vi "Create Tasks.vi"(8 "error in":errorcluster, 11 "6509 in":refnum<class "6509.lvclass">) -> (0 "error out":errorcluster, 3 "6509 out":refnum<class "6509.lvclass">)   [LabVIEW 2019, in "6509.lvlib" / "6509.lvclass"]
uses:
  Library/6509.lvclass
  C:/Users/Public/Documents/Development/builds/Instruments/Instruments.lvlibp/Library/Instruments.lvclass
  C:/Users/Public/Documents/Development/builds/Instruments/DIG_IO.lvlibp/Library/DIG_IO.lvclass
  Library/6509.lvclass/6509.ctl
  builds/Instruments/Instruments.lvlibp/Accessors/Read Resource.vi
  builds/Instruments/DIG_IO.lvlibp/Accessors/Read IO_Mode.vi
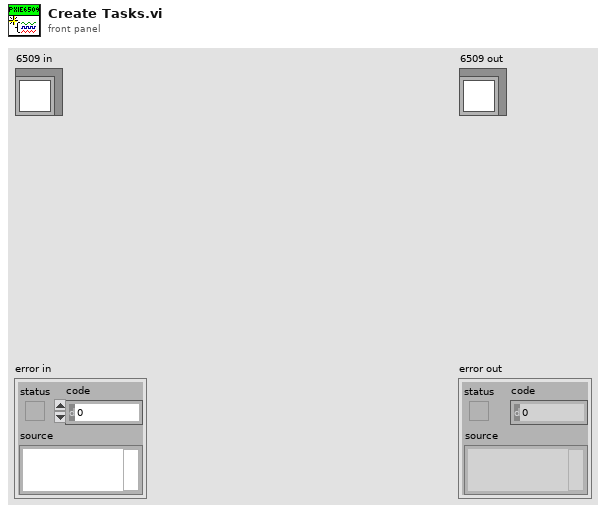
[diagram p1: front panel]
types:
  T1 = typedef "DIG_IO.lvlibp/DIG_IO.lvclass/IO Mode.ctl" = enum16{"IO", "IN", "OUT"}
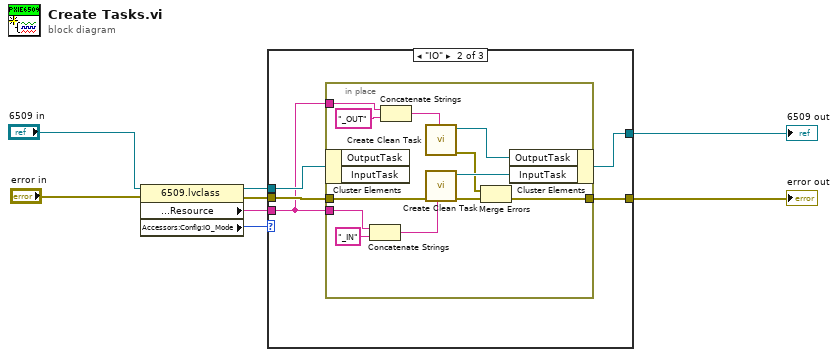
[diagram p0: block diagram]
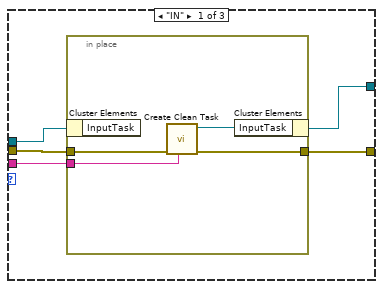
[diagram p2: hidden frame]
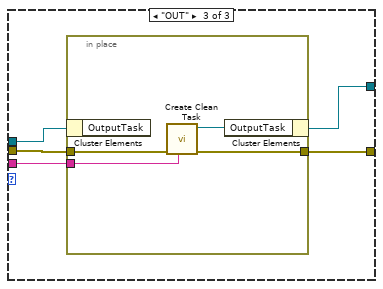
[diagram p3: hidden frame]
diagram:
  n1 = property class="6509.lvclass"(reference="6509 in", error in="error in") -> (reference out=w6:refnum<class "6509.lvclass">, error out=w4:errorcluster, "Accessors:Configuration:Resource"=w7:string, "Accessors:Config:IO_Mode"=w8:T1)
  n2 = case shown="\"IO\"" w8 {
    tunnel: w7 -> [w10 w18 w36]
    tunnel: w6 -> [w13 w22 w39]
    tunnel: [w12 w21 w38] -> w5
    tunnel: w4 -> [w11 w20 w37]
    tunnel: [w9 w19 w35] -> w3
    frame "IN" {
      n3 = in-place {
        in-place-border: w11 -> [w16]
        in-place-border: w10 -> [w15]
        in-place-border: [w14] -> w9
        n4 = in-place-cluster #1(w13) -> ()  [unwired: 1 out]
        n5 = call "Create Clean Task.vi"("Task Name"=w15, "error in (no error)"=w16) -> ("error out"=w14:errorcluster, "task out"=w17:refnum<k21>)  [unwired: 8 in]
        n6 = in-place-cluster #1("InputTask"=w17) -> (w12:refnum<class "6509.lvclass">)
      }
    }
    frame "IO" {
      n7 = in-place {
        in-place-border: w20 -> [w33]
        in-place-border: w18 -> [w32]
        in-place-border: [w25] -> w19
        in-place-border: w18 -> [w28]
        n8 = in-place-cluster #2(w22) -> ()  [unwired: 2 out]
        n9 = Concatenate Strings(w32, "_IN" ("string")) -> (w30:string)
        n10 = Concatenate Strings(w28, "_OUT" ("string")) -> (w27:string)
        n11 = call "Create Clean Task.vi"("Task Name"=w27) -> ("error out"=w23:errorcluster, "task out"=w26:refnum<k21>)  [unwired: 9 in]
        n12 = call "Create Clean Task.vi"("Task Name"=w30, "error in (no error)"=w33) -> ("error out"=w24:errorcluster, "task out"=w34:refnum<k21>)  [unwired: 8 in]
        n13 = Merge Errors(w23, w24) -> (w25:errorcluster)
        n14 = in-place-cluster #2("OutputTask"=w26, "InputTask"=w34) -> (w21:refnum<class "6509.lvclass">)
      }
    }
    frame "OUT" {
      n15 = in-place {
        in-place-border: w37 -> [w42]
        in-place-border: w36 -> [w41]
        in-place-border: [w40] -> w35
        n16 = in-place-cluster #3(w39) -> ()  [unwired: 1 out]
        n17 = call "Create Clean Task.vi"("Task Name"=w41, "error in (no error)"=w42) -> ("error out"=w40:errorcluster, "task out"=w43:refnum<k21>)  [unwired: 8 in]
        n18 = in-place-cluster #3("OutputTask"=w43) -> (w38:refnum<class "6509.lvclass">)
      }
    }
  }
  "error out" <- w3
  "6509 out" <- w5
